vi "StartData.vi"(8 "error in (no error)":errorcluster, 11 "Class In":refnum<class "PmuBase.lvclass">) -> (0 "error out":errorcluster, 3 "Class Out":refnum<class "PmuBase.lvclass">)   [LabVIEW 2018, in "SensorPlugins.lvlib" / "PmuBase.lvclass"]
uses:
  PmuBase.lvclass
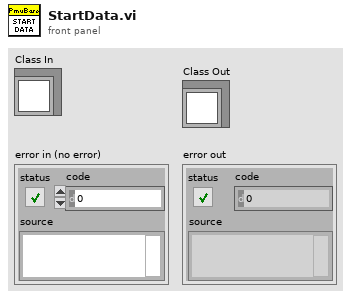
[diagram p1: front panel]
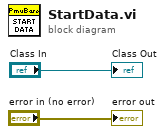
[diagram p0: block diagram]
diagram:
  "Class Out" <- "Class In"
  "error out" <- "error in (no error)"
